vi "get console output.vi"() -> (2 "console_output":string)   [LabVIEW 2019, in "libSimulationControl.lvlib"]
uses:
  libSimulationControl.lvlib
panel:
  out "error out":errorcluster
  in  "error in (no error)":errorcluster
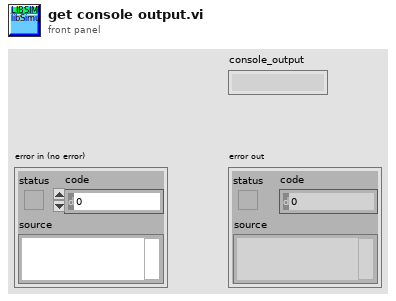
[diagram p1: front panel]
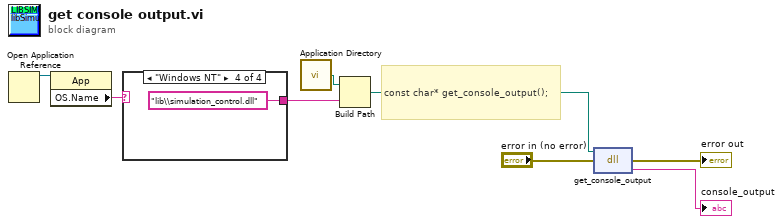
[diagram p0: block diagram]
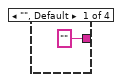
[diagram p2: hidden frame]
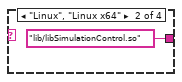
[diagram p3: hidden frame]
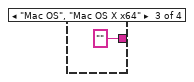
[diagram p4: hidden frame]
diagram:
  # "const char* get_console_output();"
  n1 = Open Application Reference() -> (3:w6:refnum<vi>)  [unwired: 4 in, 1 out]
  n2 = property class="App"(reference=w6) -> ("OS.Name"=w5:string)  [unwired: 1 in, 2 out]
  n3 = case shown="\"Windows NT\"" w5 {
    tunnel: ["" ("return type") "lib/libSimulationControl.so" ("name or relative path") "" ("return type") "lib\\simulation_control.dll" ("name or relative path")] -> w4
    frame "", Default {
    }
    frame "Linux", "Linux x64" {
    }
    frame "Mac OS", "Mac OS X x64" {
    }
    frame "Windows NT" {
    }
  }
  n4 = call <vilib>:"Application Directory.vi"() -> ("Application Directory"=w3:path)
  n5 = Build Path(base path=w3, name or relative path=w4) -> (appended path=w2:path)
  n6 = dll-call lib="home/paul/Schreibtisch/Biogas_plant_setup/LabView/lib/libSimulationControl.so" fn="get_console_output"(path in=w2, error in="error in (no error)") -> (error out=→"error out":errorcluster, "console_output"=→"console_output":string)  [unwired: 1 in, 1 out]
